vi "TimeToSeconds.vi"(10 "TimesMeasured":string[](array[string])) -> (2 "Seconds Passed":string[](array[string]))   [LabVIEW 2024]
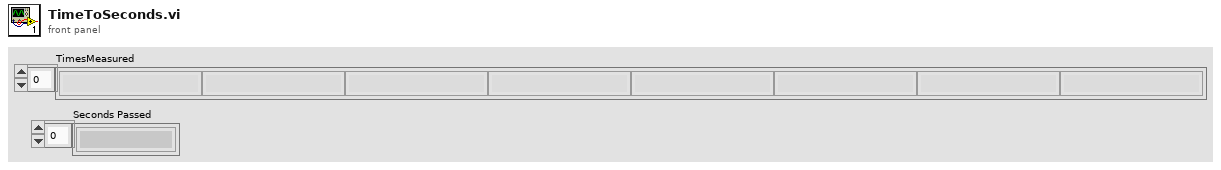
[diagram p1: front panel]
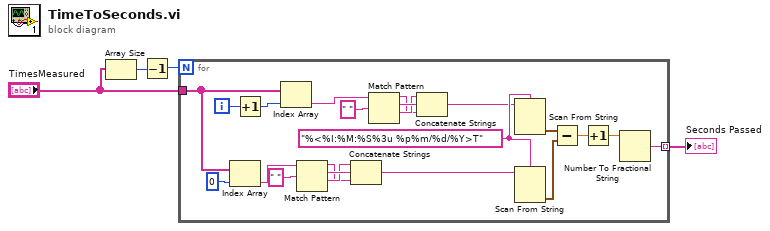
[diagram p0: block diagram]
diagram:
  n1 = Array Size(array="TimesMeasured") -> (size(s)=w3:i32)
  n2 = Decrement(x=w3) -> (x-1=w2:i32)
  n3 = for {
    N: w2 -> [_]
    tunnel: [w21] -> w1 mode=indexing
    tunnel: "TimesMeasured" -> [w26]
    i -> [w25]
    w22 = "%<%I:%M:%S%3u %p%m/%d/%Y>T" ("format string")
    n4 = Index Array(array=w26, index=0) -> (element=w12:string)
    n5 = Increment(x=w25) -> (x+1=w24:i32)
    n6 = Index Array(array=w26, index=w24) -> (element=w10:string)
    n7 = Match Pattern(string=w12, regular expression=" ") -> (before substring=w13:string, match substring=w15:string, after substring=w14:string)  [unwired: 1 in, 1 out]
    n8 = Concatenate Strings(w14, w15, w13) -> (w11:string)
    n9 = Match Pattern(string=w10, regular expression=" ") -> (before substring=w6:string, match substring=w8:string, after substring=w7:string)  [unwired: 1 in, 1 out]
    n10 = Concatenate Strings(w7, w8, w6) -> (w9:string)
    n11 = Scan From String(format string=w22, input string=w9) -> (output 1=w18:timestamp)  [unwired: 3 in, 3 out]
    n12 = Scan From String(format string=w22, input string=w11) -> (output 1=w17:timestamp)  [unwired: 3 in, 3 out]
    n13 = Subtract(x=w18, y=w17) -> (x-y=w20:dbl)
    n14 = Increment(x=w20) -> (x+1=w19:dbl)
    n15 = Number To Fractional String(number=w19) -> (F-format string=w21:string)  [unwired: 3 in]
  }
  "Seconds Passed" <- w1
